vi "D批量读取.vi"(6 "长度":i32, 8 "错误输入":errorcluster, 9 "开始":i32, 10 "数组":i32[](array[numeric]), 11 "选项":enum16{"Read", "Write"}(ring)) -> (0 "错误输出":errorcluster, 3 "D读取":T1[](array[typedef]))   [LabVIEW 2017]
uses:
  Component Assemble Input.ctl
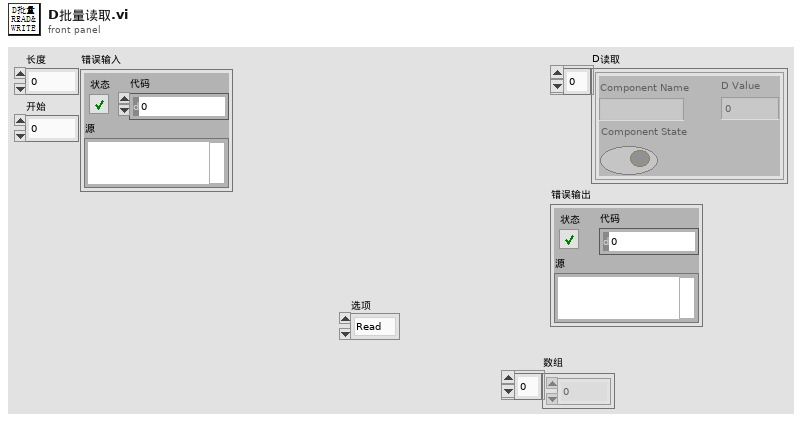
[diagram p1: front panel]
types:
  T1 = typedef "Component Assemble Input.ctl" = cluster{"Component Name":string, "Component State":bool, "D Value":i32}
  T2 = typedef "MX操作选项.ctl" = enum16{"MX Initial ", "MX Close", "X&Y&M Read", "X&Y&M Write", "D Read", "D Write", "Many component Read", "Many component Write", "Load Function Global"}
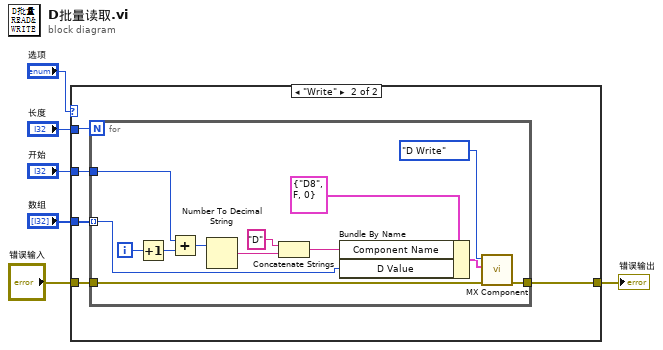
[diagram p0: block diagram]
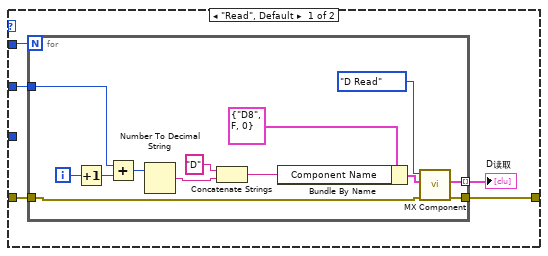
[diagram p2: hidden frame]
diagram:
  n1 = case shown="\"Write\"" "选项" {
    tunnel: "长度" -> [w11 w29]
    tunnel: "开始" -> [w10 w28]
    tunnel: "数组" -> [_ w27]
    tunnel: [w8 w26] -> w2
    tunnel: "错误输入" -> [w7 w25]
    frame "Read", Default {
      n2 = for {
        N: w11 -> [_]
        tunnel: w7 -> [w23]
        tunnel: [w15] -> w9 mode=indexing
        tunnel: w10 -> [w13]
        tunnel: [w12] -> w8
        i -> [w20]
        n3 = Increment(x=w20) -> (x+1=w19:i32)
        n4 = Add(x=w13, y=w19) -> (x+y=w14:i32)
        n5 = Number To Decimal String(number=w14) -> (decimal integer string=w18:string)  [unwired: 1 in]
        n6 = Concatenate Strings("D" ("字符串"), w18) -> (w17:string)
        n7 = Bundle By Name(cluster=T1 {"Component Name"="D8", "Component State"=FALSE, "D Value"=0} ("Component Assemble Input"), "Component Name"=w17) -> (w16:T1)
        n8 = call "MX Component.vi"("错误输入"=w23, "Component Assemble Input"=w16, "MX操作选项"=MX操作选项."D Read") -> ("错误输出"=w12:errorcluster, "Component Assemble Output"=w15:T1)  [unwired: 6 in, 1 out]
      }
      "D读取" <- w9
    }
    frame "Write" {
      n9 = for {
        N: w29 -> [_]
        tunnel: w25 -> [w41]
        tunnel: w28 -> [w32]
        tunnel: w27 -> [w31] mode=indexing
        tunnel: [w30] -> w26
        i -> [w38]
        n10 = Increment(x=w38) -> (x+1=w37:i32)
        n11 = Add(x=w32, y=w37) -> (x+y=w33:i32)
        n12 = Number To Decimal String(number=w33) -> (decimal integer string=w36:string)  [unwired: 1 in]
        n13 = Concatenate Strings("D" ("字符串"), w36) -> (w35:string)
        n14 = Bundle By Name(cluster=T1 {"Component Name"="D8", "Component State"=FALSE, "D Value"=0} ("Component Assemble Input"), "Component Name"=w35, "D Value"=w31) -> (w34:T1)
        n15 = call "MX Component.vi"("错误输入"=w41, "Component Assemble Input"=w34, "MX操作选项"=MX操作选项."D Write") -> ("错误输出"=w30:errorcluster)  [unwired: 6 in, 2 out]
      }
    }
  }
  "错误输出" <- w2
